vi "set_config_cluster.vi"(8 "error in (no error)":errorcluster, 10 "config cluster variant":variant, 11 "ScanHeadDL090202 in":refnum<class "ScanHeadDL090202.lvclass">) -> (0 "error out":errorcluster, 3 "ScanHeadDL090202 out":refnum<class "ScanHeadDL090202.lvclass">)   [LabVIEW 2010, in "ScanHeadDL090202.lvclass"]
uses:
  ScanHeadDL090202.lvclass
  ScanHeadDL090202.lvclass/ScanHeadDL090202.ctl
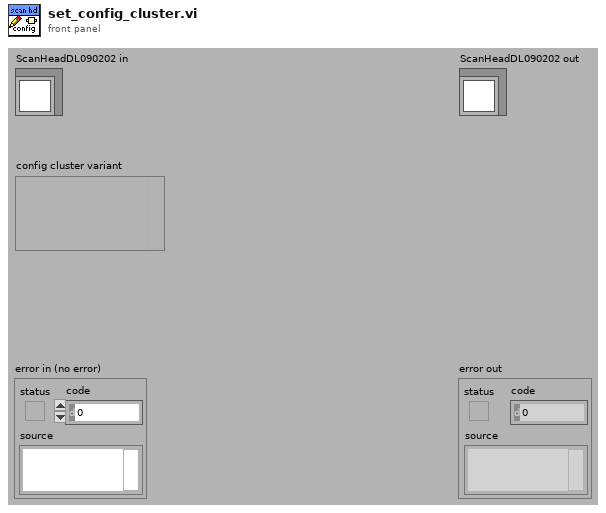
[diagram p1: front panel]
types:
  T1 = typedef "ScanHeadDL090202.lvclass/config_data_cluster.ctl" = cluster{"subcomponents":T2, "scanner factors":dbl[unit][], "modifier factor":dbl, "update frequency":dbl[unit], "LSID":T4, "visibility":cluster{"Zoom":bool, "RotateX":bool, "RotateY":bool, "TranslateX":bool, "TranslateY":bool, "TranslateZ":bool}, "position channel indices (x/y/z)":i32[], "available settings":T5[], "default settings":string}
  T2 = typedef "ScanHeadDL090202.lvclass/subcomponent_specifications_cluster.ctl" = cluster{"scanners":T3[], "intensity modifier":T3, "clock":T3, "shutter":T3}
  T3 = typedef "plugin_specification.ctl" = cluster{"class path":string, "configuration":string, "label":string, "settings name":string}
  T4 = typedef "LSID_cluster.ctl" = cluster{"identifier":string, "revision":i32}
  T5 = typedef "settings_specification_cluster.ctl" = cluster{"name":string, "label":string}
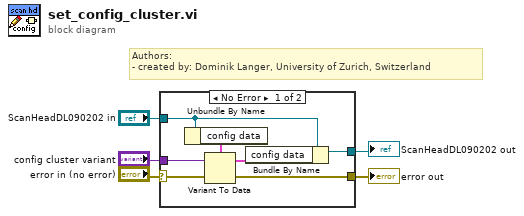
[diagram p0: block diagram]
diagram:
  # "Authors: \n- created by: Dominik Langer, University of Zurich, Switzerland"
  n1 = case shown="No Error" "error in (no error)" {
    selector: "error in (no error)" -> [w10 w14]
    tunnel: "ScanHeadDL090202 in" -> [w8 w13]
    tunnel: [w7 w13] -> w2
    tunnel: [w6 w14] -> w1
    tunnel: "config cluster variant" -> [w11 _]
    frame No Error {
      n2 = Unbundle By Name(w8) -> ("config data"=w12:T1)
      n3 = Variant To Data(error in=w10, Variant=w11, type=w12) -> (error out=w6:errorcluster, data=w9:T1)
      n4 = Bundle By Name(cluster=w8, "config data"=w9) -> (w7:refnum<class "ScanHeadDL090202.lvclass">)
    }
    frame Error {
    }
  }
  "error out" <- w1
  "ScanHeadDL090202 out" <- w2
